vi "TSM DMM Pins to Sessions.vi"(0 "TSM Context":T2, 5 "Pins":tag[](array[tag]), 11 "error in":errorcluster) -> (4 "DMM TSM Out":T1, 15 "error out":errorcluster)   [LabVIEW 2020]
doc: "Populates the TSM DMM cluster for the specified pin(s) and pin group(s)."
uses:
  <vilib>/NI_TestStand_SemiconductorModule/NI_TestStand_Semiconductor_Module.lvlibp/PinMap/General/SemiconductorModuleContext.ctl
  TSM DMM.ctl
  <vilib>/NI_TestStand_SemiconductorModule/NI_TestStand_Semiconductor_Module.lvlibp/PinMap/PinQueryContext/MultiplePinMultipleSessionQueryContext/MultiplePinMultipleSessionQueryContext.lvclass
  <vilib>/NI_TestStand_SemiconductorModule/NI_TestStand_Semiconductor_Module.lvlibp/PinMap/DMM/PinsToNIDMMSessions.vi
  <vilib>/NI_TestStand_SemiconductorModule/NI_TestStand_Semiconductor_Module.lvlibp
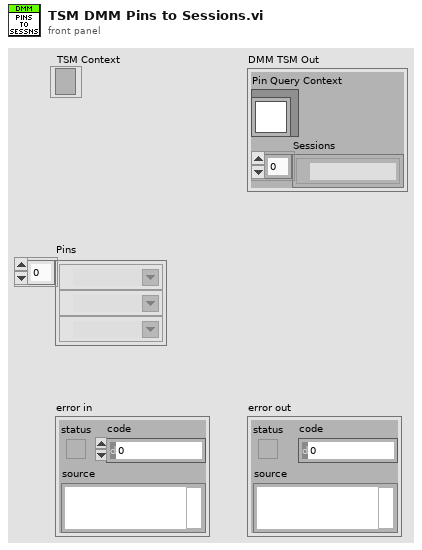
[diagram p1: front panel]
types:
  T1 = typedef "TSM DMM.ctl" = cluster{"Pin Query Context":refnum<class "MultiplePinMultipleSessionQueryContext.lvclass">, "Sessions":refnum<k15>[]}
  T2 = typedef "NI_TestStand_Semiconductor_Module.lvlibp/SemiconductorModuleContext.ctl" = refnum<k7>
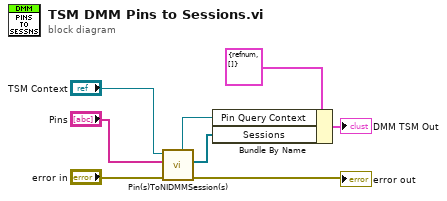
[diagram p0: block diagram]
diagram:
  n1 = call-poly <vilib>:"Pin(s)ToNIDMMSession(s).vi"("error in (no error)"="error in", "Pins"="Pins", "Semiconductor Module Context"="TSM Context") -> ("error out"=→"error out":errorcluster, "Instrument Sessions"=w3:refnum<k15>[], "Pin Query Context"=w4:refnum<class "MultiplePinMultipleSessionQueryContext.lvclass">)  [unwired: 5 in, 1 out]
  n2 = Bundle By Name(cluster=T1 {"Pin Query Context"=refnum, "Sessions"=[]} ("DMM TSM"), "Pin Query Context"=w4, "Sessions"=w3) -> (→"DMM TSM Out":T1)
